vi "Read Transconductance (Current).vi"(0 "VISA resource name":refnum<visa-resource-name>, 1 "Pulse Stop Level (0.1 A)":dbl=0.1, 2 "Pulse Start Level (0 A)":dbl, 5 "Source Measure Unit Channel (0: Channel A)":i32(ring) items=["Channel A", "Channel B"], 7 "Current Buffer (ibuffer)":string="ibuffer", 9 "Voltage Buffer (vbuffer)":string="vbuffer", 11 "error in (no error)":errorcluster, 12 "Pulse Measure Cycles (10)":i32=10) -> (4 "VISA resource name out":refnum<visa-resource-name>, 6 "Transconductance":dbl[](array[numeric]), 8 "Current (A)":dbl[](array[numeric]), 10 "Voltage (V)":dbl[](array[numeric]), 15 "error out":errorcluster)   [LabVIEW 2020, in "Keithley 2600 Series.lvlib"]
doc: "Performs a linear current sweep and calculates the transconductance.\n\n<b>Note:</b>\nThere are three options for the measurements during the current sweep: transconductance measurement; transconductance and voltage measurement; transconductance, voltage and current measurement."
uses:
  <instrlib>/Keithley 2600 Series/Keithley 2600 Series.lvlib
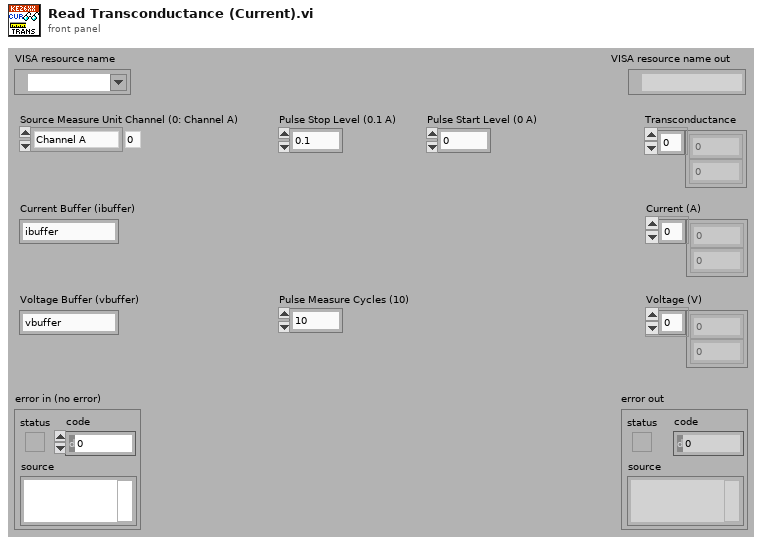
[diagram p1: front panel]
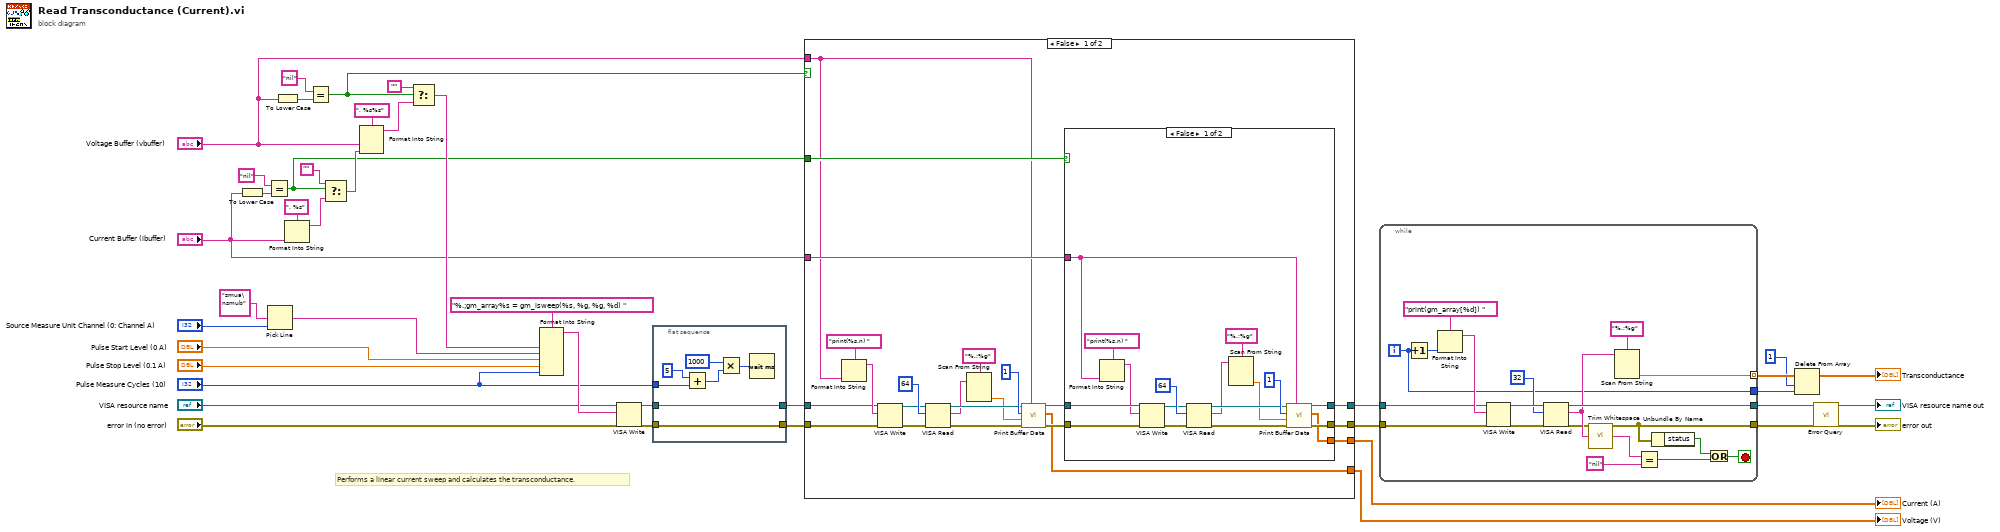
[diagram p0: block diagram]
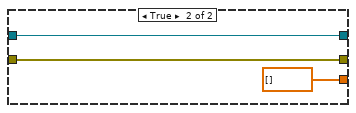
[diagram p2: hidden frame]
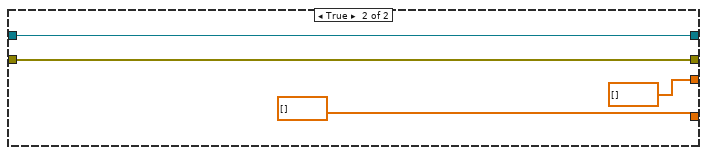
[diagram p3: hidden frame]
diagram:
  # "Performs a linear current sweep and calculates the transconductance."
  n1 = To Lower Case(string="Current Buffer (ibuffer)") -> (all lower case string=w9:string)
  n2 = Equal?(x="nil", y=w9) -> (x = y?=w20:bool)
  n3 = Pick Line(multi-line string="smua\nsmub", line index="Source Measure Unit Channel (0: Channel A)") -> (output string=w24:string)  [unwired: 1 in]
  n4 = To Lower Case(string="Voltage Buffer (vbuffer)") -> (all lower case string=w11:string)
  n5 = Format Into String(format string=", %s", "Current Buffer (ibuffer)") -> (resulting string=w28:string)  [unwired: 2 in, 1 out]
  n6 = Equal?(x="nil", y=w11) -> (x = y?=w21:bool)
  n7 = Select(t="", s=w20, f=w28) -> (s? t:f=w27:string)
  n8 = Format Into String(format string=", %s%s", "Voltage Buffer (vbuffer)", w27) -> (resulting string=w26:string)  [unwired: 2 in, 1 out]
  n9 = Select(t="", s=w21, f=w26) -> (s? t:f=w25:string)
  n10 = Format Into String(format string="%.;gm_array%s = gm_isweep(%s, %g, %g, %d) ", w25, w24, "Pulse Start Level (0 A)", "Pulse Stop Level (0.1 A)", "Pulse Measure Cycles (10)") -> (resulting string=w41:string)  [unwired: 2 in, 1 out]
  n11 = VISA Write(VISA resource name="VISA resource name", write buffer=w41, error in (no error)="error in (no error)") -> (VISA resource name out=w13:refnum<visa-resource-name>, error out=w12:errorcluster)  [unwired: 1 out]
  n12 = flat-sequence {
    tunnel: w13 -> [w43]
    tunnel: w12 -> [w49]
    tunnel: [w49] -> w2
    tunnel: "Pulse Measure Cycles (10)" -> [w44]
    tunnel: [w43] -> w1
    frame #0 {
      n13 = Add(x=5, y=w44) -> (x+y=w46:i32)
      n14 = Multiply(x=1000 ("y"), y=w46) -> (x*y=w45:i32)
      n15 = Wait (ms)(milliseconds to wait=w45) -> ()  [unwired: 1 out]
    }
  }
  n16 = case shown="False" w21 {
    tunnel: [w56 w95] -> w17
    tunnel: w1 -> [w60 w95]
    tunnel: w2 -> [w59 w94]
    tunnel: [w55 w94] -> w16
    tunnel: w20 -> [w54 _]
    tunnel: "Current Buffer (ibuffer)" -> [w53 _]
    tunnel: [w52 dbl[] [] ("Buffer Data")] -> w19
    tunnel: [w51 dbl[] [] ("Buffer Data")] -> w18
    tunnel: "Voltage Buffer (vbuffer)" -> [w50 _]
    frame False {
      n17 = Format Into String(format string="print(%s.n) ", w50) -> (resulting string=w61:string)  [unwired: 2 in, 1 out]
      n18 = VISA Write(VISA resource name=w60, write buffer=w61, error in (no error)=w59) -> (VISA resource name out=w64:refnum<visa-resource-name>, error out=w63:errorcluster)  [unwired: 1 out]
      n19 = VISA Read(VISA resource name=w64, byte count=u32 64, error in (no error)=w63) -> (VISA resource name out=w69:refnum<visa-resource-name>, read buffer=w67:string, error out=w68:errorcluster)  [unwired: 1 out]
      n20 = Scan From String(format string="%.;%g", input string=w67) -> (output 1=w66:dbl)  [unwired: 3 in, 3 out]
      n21 = call <instrlib>:"Print Buffer Data.vi"("Reading Buffer (smua.nvbuffer1)"=w50, "error in (no error)"=w68, "End Index (1)"=w66, "Start Index (1)"=1 ("Start Index (0)"), "VISA resource name"=w69) -> ("error out"=w57:errorcluster, "Buffer Data"=w52:dbl[], "VISA resource name out"=w58:refnum<visa-resource-name>)  [unwired: 4 in]
      n22 = case shown="False" w54 {
        tunnel: w58 -> [w80 w91]
        tunnel: w57 -> [w79 w90]
        tunnel: [w78 w91] -> w56
        tunnel: [w77 w90] -> w55
        tunnel: w53 -> [w74 _]
        tunnel: [w73 dbl[] [] ("Buffer Data")] -> w51
        frame False {
          n23 = Format Into String(format string="print(%s.n) ", w74) -> (resulting string=w75:string)  [unwired: 2 in, 1 out]
          n24 = VISA Write(VISA resource name=w80, write buffer=w75, error in (no error)=w79) -> (VISA resource name out=w82:refnum<visa-resource-name>, error out=w81:errorcluster)  [unwired: 1 out]
          n25 = VISA Read(VISA resource name=w82, byte count=u32 64, error in (no error)=w81) -> (VISA resource name out=w86:refnum<visa-resource-name>, read buffer=w84:string, error out=w85:errorcluster)  [unwired: 1 out]
          n26 = Scan From String(format string="%.;%g", input string=w84) -> (output 1=w83:dbl)  [unwired: 3 in, 3 out]
          n27 = call <instrlib>:"Print Buffer Data.vi"("Reading Buffer (smua.nvbuffer1)"=w74, "error in (no error)"=w85, "End Index (1)"=w83, "Start Index (1)"=1 ("Start Index (0)"), "VISA resource name"=w86) -> ("error out"=w77:errorcluster, "Buffer Data"=w73:dbl[], "VISA resource name out"=w78:refnum<visa-resource-name>)  [unwired: 4 in]
        }
        frame True {
        }
      }
    }
    frame True {
    }
  }
  "Voltage (V)" <- w19
  "Current (A)" <- w18
  n28 = while {
    tunnel: w17 -> [w111]
    tunnel: w16 -> [w110]
    tunnel: [w107] -> w15
    tunnel: [w99] -> w14
    tunnel: [w101] -> w7 mode=indexing
    tunnel: [w100] -> w5
    i -> [w100]
    stop <- w98 stop-if-true
    n29 = Increment(x=w100) -> (x+1=w114:i32)
    n30 = Format Into String(format string="print(gm_array[%d]) ", w114) -> (resulting string=w112:string)  [unwired: 2 in, 1 out]
    n31 = VISA Write(VISA resource name=w111, write buffer=w112, error in (no error)=w110) -> (VISA resource name out=w109:refnum<visa-resource-name>, error out=w108:errorcluster)  [unwired: 1 out]
    n32 = VISA Read(VISA resource name=w109, byte count=u32 32, error in (no error)=w108) -> (VISA resource name out=w107:refnum<visa-resource-name>, read buffer=w103:string, error out=w99:errorcluster)  [unwired: 1 out]
    n33 = call <vilib>:"Trim Whitespace.vi"("string"=w103) -> ("trimmed string"=w104:string)  [unwired: 1 in]
    n34 = Scan From String(format string="%.;%g", input string=w103) -> (output 1=w101:dbl)  [unwired: 3 in, 3 out]
    n35 = Equal?(x=w104, y="nil") -> (x = y?=w96:bool)
    n36 = Unbundle By Name(w99) -> ("status"=w97:bool)
    n37 = Or(x=w97, y=w96) -> (x .or. y?=w98:bool)
  }
  n38 = Delete From Array(array=w7, length=1, index=w5) -> (array with subset deleted=→"Transconductance":dbl[])  [unwired: 1 out]
  n39 = call <instrlib>:"Error Query.vi"("error in (no error)"=w14, "VISA resource name"=w15) -> ("error out"=→"error out":errorcluster, "VISA resource name out"=→"VISA resource name out":refnum<visa-resource-name>)  [unwired: 6 in, 2 out]
